vi "Cfg PopUp _ Registration.vi"(7 "PopUp":string, 8 "error in":errorcluster caption="错误输入", 10 "ColTypes[ ]":T1[](array[typedef]), 11 "Ref.Tree":refnum<vi>) -> (0 "error out":errorcluster caption="错误输出")   [LabVIEW 2016]
uses:
  ToolKit/Popup/Private/Ctrls/POP_Popup Call Parameters.ctl
  ToolKit/Popup/Private/Ctrls/POP_Data Type.ctl
  <vilib>/Utility/miscctls.llb/LVBrowseOptionsTypeDef.ctl
  HardWare/Ctrls/HardWare _ Channel Configurations PopUp Type.ctl
panel:
  in  "PopupStr":T3={"Prop Type"=enum."Unkown", "Initial Value"=variant, "Caption Strings"=[], "Ring Strings"=[], "Cell Rect"={"left"=0, "top"=0, "right"=0, "bottom"=0}, "Mouse Coords"={"x"=0, "y"=0}, "Call Data"=variant, "Ring Values"=[], "Browse Options"={"Prompt"="", "Match Pattern"="", "Mode"=enum."existing file", "Start Path"=path "", "Pattern Label"="", "Button Text"=""}, "Combo Box"={"Allow Undefined Strings"=FALSE}}
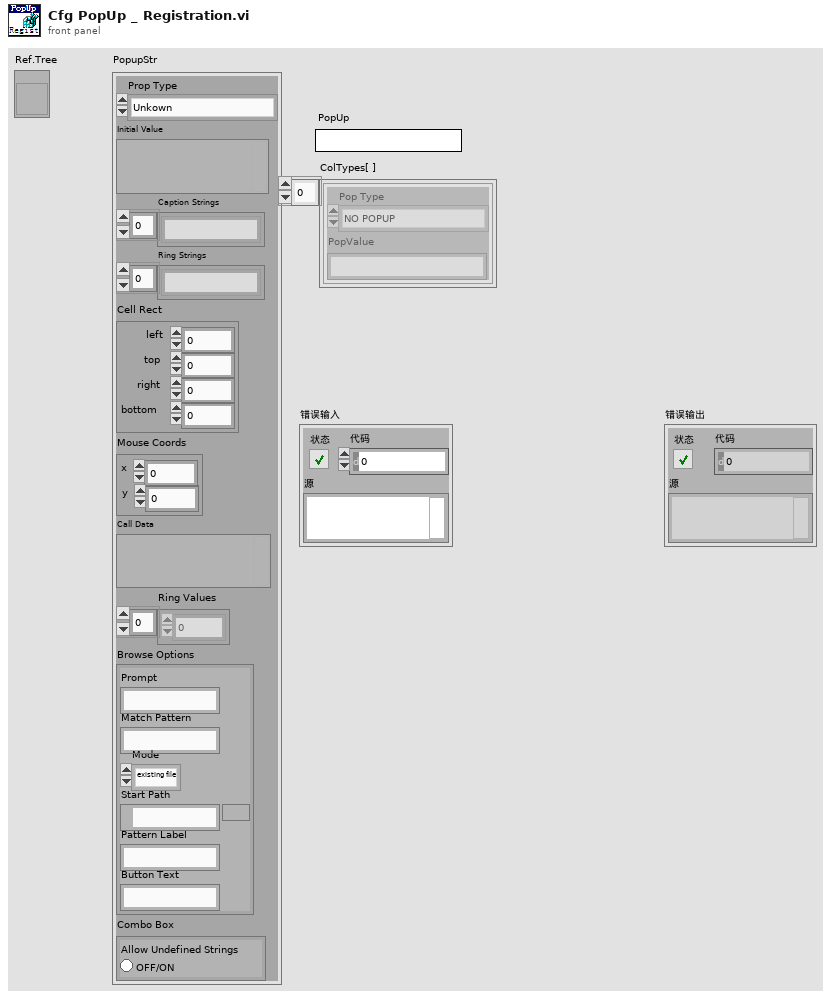
[diagram p1: front panel]
types:
  T1 = typedef "HardWare _ Channel Configurations PopUp Type.ctl" = cluster{"Pop Type":T2, "PopValue":string}
  T2 = typedef "POP_Data Type.ctl" = enum16{"NO POPUP", "Unkown", "String", "Integer", "Float", "Color", "Boolean", "Ring", "Captioned String", "Captioned Integer", "Button Color", "2 Int Cluster", "4 Int Cluster", "6-Dbl Cluster", "Path", "Combox", "Time", "ShotCut String"}
  T3 = typedef "POP_Popup Call Parameters.ctl" = cluster{"Prop Type":T2, "Initial Value":variant, "Caption Strings":string[], "Ring Strings":string[], "Cell Rect":cluster{"left":i16, "top":i16, "right":i16, "bottom":i16}, "Mouse Coords":cluster{"x":i16, "y":i16}, "Call Data":variant, "Ring Values":ext[], "Browse Options":T4, "Combo Box":cluster{"Allow Undefined Strings":bool}}
  T4 = typedef "LVBrowseOptionsTypeDef.ctl" = cluster{"Prompt":string, "Match Pattern":string, "Mode":enum32{"existing file", "new file", "new or existing file", "existing dir", "new dir", "new or existing dir", "existing file (use LLBs)", "new file (use LLBs)", "new or existing file (use LLBs)", "new or existing file or directory (use LLBs)", "existing dir (use LLBs)", "new dir (use LLBs)", "new or existing dir (use LLBs)", "existing file or dir", "new file or dir", "new or existing file or dir", "existing file or dir (use LLBs)", "new file or dir (use LLBs)"}, "Start Path":path, "Pattern Label":string, "Button Text":string}
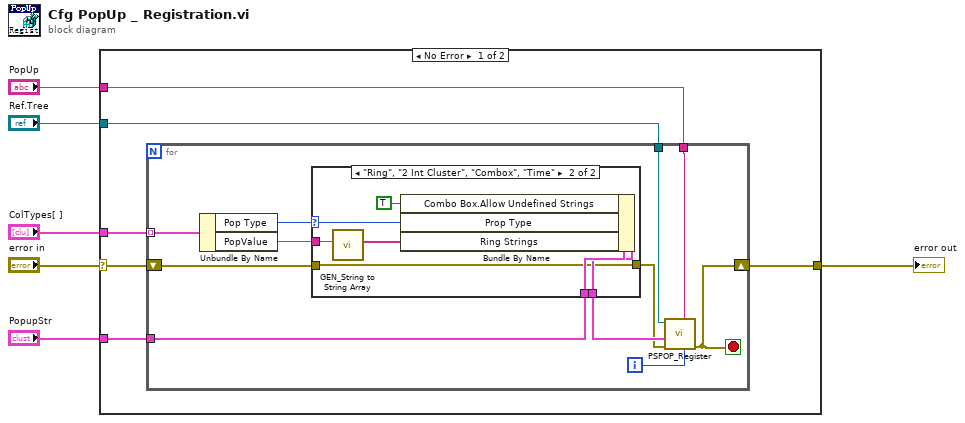
[diagram p0: block diagram]
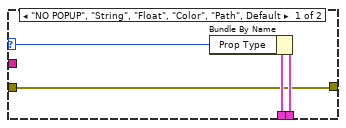
[diagram p2: hidden frame]
diagram:
  n1 = case shown="No Error" "error in" {
    selector: "error in" -> [w11 w35]
    tunnel: [w9 w35] -> w5
    tunnel: "Ref.Tree" -> [w8 _]
    tunnel: "PopUp" -> [w12 _]
    tunnel: "PopupStr" -> [w10 _]
    tunnel: "ColTypes[ ]" -> [w7 _]
    frame No Error {
      n2 = for {
        tunnel: w12 -> [w18]
        tunnel: w10 -> [w22]
        shift-right: [w17] -> w9
        shift-left: w11 -> [w20]
        tunnel: w8 -> [w16]
        tunnel: w7 -> [w15] mode=indexing
        i -> [w23]
        stop <- w17 stop-if-true
        n3 = Unbundle By Name(w15) -> ("Pop Type"=w14:T2, "PopValue"=w13:string)
        n4 = case shown="\"Ring\", \"2 Int Cluster\", \"Combox\", \"Time\"" w14 {
          selector: w14 -> [w25 w32]
          tunnel: w22 -> [w27 w34]
          tunnel: [w26 w33] -> w21
          tunnel: w13 -> [_ w30]
          tunnel: w20 -> [w24 w31]
          tunnel: [w24 w31] -> w19
          frame "NO POPUP", "String", "Float", "Color", "Path", Default {
            n5 = Bundle By Name(cluster=w27, "Prop Type"=w25) -> (w26:T3)
          }
          frame "Ring", "2 Int Cluster", "Combox", "Time" {
            n6 = call "GEN_String to String Array.vi"("String in"=w30) -> ("String Array out"=w29:string[])  [unwired: 10 in]
            n7 = Bundle By Name(cluster=w34, "Combo Box.Allow Undefined Strings"=TRUE, "Prop Type"=w32, "Ring Strings"=w29) -> (w33:T3)
          }
        }
        n8 = call "PSPOP_Register.vi"("Col (unwired = all columns)"=w23, "Name"=w18, "error in (no error)"=w19, "Parameters"=w21, "Ctl Refnum"=w16) -> ("error out"=w17:errorcluster)  [unwired: 5 in, 1 out]
      }
    }
    frame Error {
    }
  }
  "error out" <- w5
